vi "Read headers.vi"(8 "error in (no error)":errorcluster, 11 "httpHeaders in":refnum<class "httpHeaders.lvclass">) -> (0 "error out":errorcluster, 2 "headers":cluster{"header":string, "value":string}[](array[cluster]), 3 "httpHeaders out":refnum<class "httpHeaders.lvclass">)   [LabVIEW 2020, in "httpClient.lvlib" / "httpHeaders.lvclass"]
uses:
  httpHeaders.lvclass
  httpHeaders.lvclass/httpHeaders.ctl
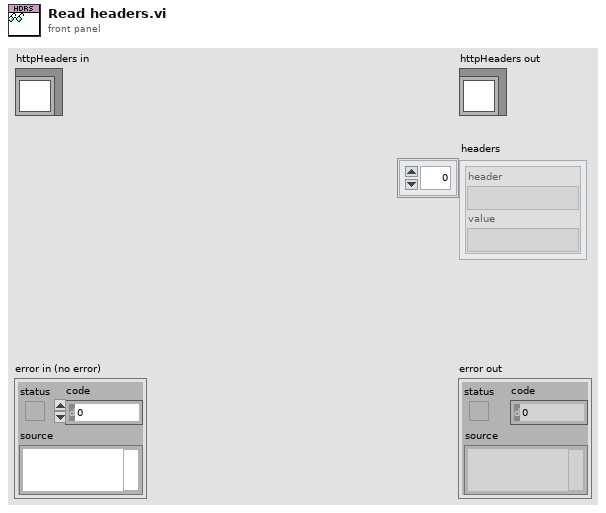
[diagram p1: front panel]
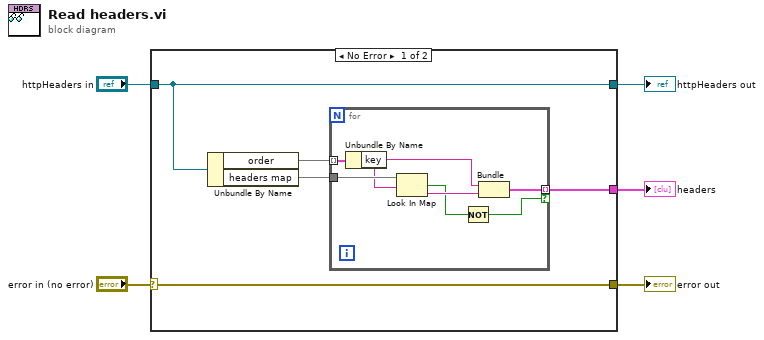
[diagram p0: block diagram]
diagram:
  n1 = case shown="No Error" "error in (no error)" {
    selector: "error in (no error)" -> [w10 w18]
    tunnel: [w10 w18] -> w4
    tunnel: [w9 w19] -> w2
    tunnel: "httpHeaders in" -> [w9 w19]
    tunnel: [w6 _] -> w1
    frame No Error {
      n2 = Unbundle By Name(w9) -> ("order"=w7:map{i32, string}, "headers map"=w8:map{string, string})
      n3 = for {
        tunnel: w8 -> [w17]
        tunnel: w7 -> [w16] mode=indexing
        tunnel: [w13] -> w6 mode=indexing if=w11
        n4 = Unbundle By Name(w16) -> ("key"=w15:string)
        n5 = Look In Map(map=w17, key=w15) -> (key not found?=w12:bool, value=w14:string)  [unwired: 1 in]
        n6 = Not(x=w12) -> (.not. x?=w11:bool)
        n7 = Bundle("key"=w15, "value"=w14) -> (w13:cluster{"key":string, "value":string})  [unwired: 1 in]
      }
    }
    frame Error {
    }
  }
  "error out" <- w4
  "httpHeaders out" <- w2
  "headers" <- w1
